vi "stringArrayInput.vi"() -> ()   [LabVIEW 2017]
panel:
  in  "Stop Button":bool
  out "sorted array":string[](array[string])
  in  "Array":string[](array[string])
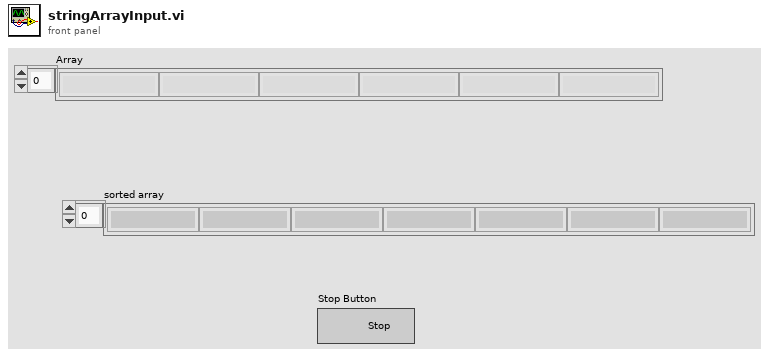
[diagram p1: front panel]
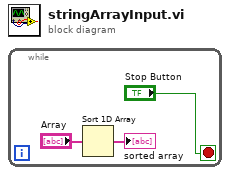
[diagram p0: block diagram]
diagram:
  n1 = while {
    stop <- "Stop Button" stop-if-true
    n2 = Sort 1D Array(array="Array") -> (sorted array=→"sorted array":string[])
  }
